vi "PadBoardWithBlock.vi"(11 "Board":T1[][](array[typedef])) -> (3 "appended array":T1[][](array[typedef]))   [LabVIEW 2015, in "TronviewGame.lvlib"]
uses:
  TronviewGame.lvlib
  Board/FieldState.ctl
  Board/Board.lvclass
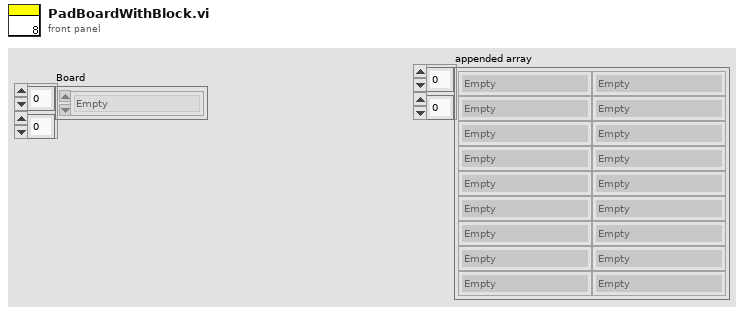
[diagram p1: front panel]
types:
  T1 = typedef "TronviewGame.lvlib/Board.lvclass/FieldState.ctl" = enum16{"Empty", "Blocked", "Player1Position", "Player2Postion", "Player1Marked", "Player2Marked"}
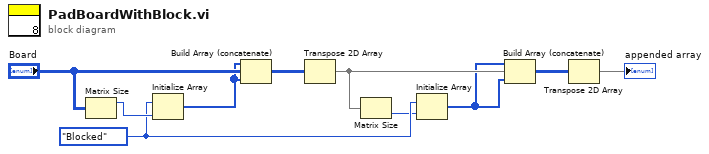
[diagram p0: block diagram]
diagram:
  w4 = FieldState."Blocked" ("FieldState")
  n1 = Matrix Size(0:"Board") -> (1:w9:i32)  [unwired: 1 out]
  n2 = Initialize Array(w4, w9) -> (w7:T1[])
  n3 = Build Array (concatenate)(w7, "Board", w7) -> (w8:T1[][])
  n4 = Transpose 2D Array(2D array=w8) -> (transposed array=w3:T1[][])
  n5 = Matrix Size(0:w3) -> (2:w1:i32)  [unwired: 1 out]
  n6 = Initialize Array(w4, w1) -> (w2:T1[])
  n7 = Build Array (concatenate)(w2, w3, w2) -> (w6:T1[][])
  n8 = Transpose 2D Array(2D array=w6) -> (transposed array=→"appended array":T1[][])
